vi "Function.vi"(8 "error in (no error)":errorcluster, 9 "B":T1, 10 "A":T1, 11 "OR in":refnum<class "NOR_Bool.lvclass">) -> (0 "error out":errorcluster, 2 "Result":T1, 3 "OR out":refnum<class "NOR_Bool.lvclass">)   [LabVIEW 2021, in "NOR_Bool.lvclass"]
uses:
  NOR_Bool.lvclass
  Type.ctl
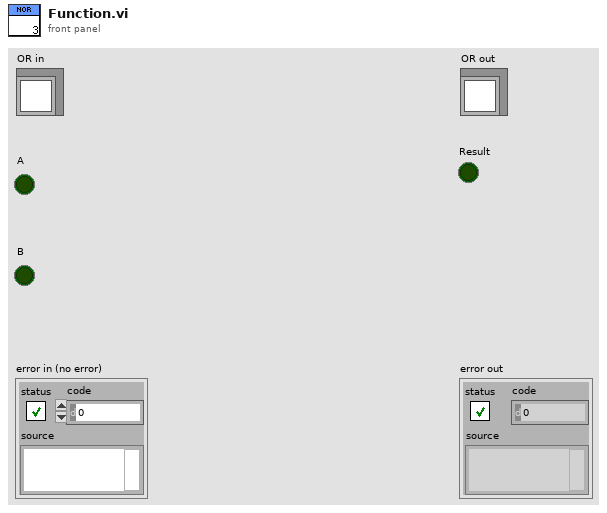
[diagram p1: front panel]
types:
  T1 = typedef "NOR_Bool.lvclass/Type.ctl" = bool
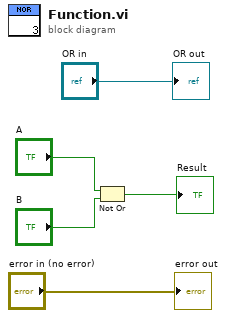
[diagram p0: block diagram]
diagram:
  n1 = Not Or(1:"B", 2:"A") -> (0:→"Result":T1)
  "error out" <- "error in (no error)"
  "OR out" <- "OR in"
